vi "ecg_ncs_v2_2Prod_1Cons.vi"() -> ()   [LabVIEW 2016]
uses:
  <instrlib>/niUSRP/niUSRP Timestamp.ctl
  C:/Program Files/National Instruments/LabVIEW 2016/examples/Instrument IO/Serial/support/Serial - Settings.ctl
  <vilib>/Analysis/coordinate.llb/Wrap Angle (array).vi
  <instrlib>/niUSRP/niUSRP Configure Time Start Trigger.vi
  <vilib>/Instr/_visa.llb/VISA Configure Serial Port (Instr).vi
  <vilib>/Analysis/3filter.llb/Butterworth Filter (DBL).vi
  <instrlib>/niUSRP/niUSRP Write Tx Data (2D CDB).vi
  <instrlib>/niUSRP/niUSRP Fetch Rx Data (2D CDB).vi
  <vilib>/measure/NI_MABase.lvlib
  <vilib>/Analysis/NI_AALBase.lvlib
  <vilib>/Analysis/NI_AALPro.lvlib
  <vilib>/Analysis/NI_AAL_Angle.lvlib
panel:
  in  "timeout in ms (-1)":i32=1
  out "size(s) 3":i32
  out "size(s) 2":i32
  out "Serial Settings:Number of Bytes at Serial Port":u32
  in  "Stop":bool
  out "Poor Sensor Quality: \nSensor off":bool
  out "Poor Sensor Quality: \nSensor on":bool
  out "Heart Rate 2":u16[](array[numeric])
  out "Stop Loop":bool=TRUE
  out "Loop index":i32
  out "size(s)":i32
  in  "Read Count":u32=80
  out "return count":u32=24
  in  "Serial Settings":T1={"baud rate"=57600, "data bits"=8, "parity"=enum."None", "stop bits"=10, "flow control"=0} {"flow control" items=["None"=0, "XON/XOFF"=1, "RTS/CTS"=2, "DTR/DSR"=4]; "stop bits" items=["1.0"=10, "1.5"=15, "2.0"=20]; "data bits" min=5 max=8 step=1; "baud rate" items=["75"=75, "110"=110, "134"=134, "150"=150, "300"=300, "600"=600, "1200"=1200, "1800"=1800, "2400"=2400, "4800"=4800, "7200"=7200, "9600"=9600, "14400"=14400, "19200"=19200, "28800"=28800, "38400"=38400, "56000"=56000, "57600"=57600, "115200"=115200, "128000"=128000, "230400"=230400]}
  in  "VISA resource name":refnum<visa-resource-name>="bmd101"
  in  "?":enum32{"ECG", "Heart Rate"}(tab)
  out "?":i16(graph)=106
  out "?":u8[](graph)
  in  "File Name":string="Test"
  in  "order1":i32=5
  in  "Path":path=path "D:/Research/SummerFall17Spring18/CnC/NCS/EcgNcsCorrelation"
  in  "Low-Pass Freq":dbl=200.0 format="%#_13g"
  in  "Sampling Rate":i32=512
  out "Gain":dbl=-15.0
  out "Bandwidth":dbl=56000000.0
  out "Coerced Carrier Frequency":dbl=2000000000.0 format="%#.17g"
  out "Coerced Tx IQ rate":dbl=992969.6965345087
  out "Coerced Rx IQ rate":dbl=1023999.9995512121
  out "error IO":errorcluster={"status"=FALSE, "code"=-1074118647, "source"=""}
  in  "Rx Number of Samples":i32=2000
  in  "Tab Control 2":enum32{"NI-294x/295x", "NI-2900/2901"}(tab)=enum."NI-2900/2901"
  in  "channel 0 carrier\n frequency [Hz]":dbl=2000000000.0 format="%#_6p"
  in  "Rx carrier frequency [Hz]":dbl=2000000000.0 format="%#_6p"
  in  "Tx carrier frequency [Hz]":dbl=1000000000.0 format="%#_6p"
  in  "Start Trigger Time":T2={"whole seconds"=1, "fractional seconds"=0.0}
  out "Tx Active Antenna":string="TX1"
  in  "Tab Control":T3(tab)=enum."Tx"
  out "NCS tag Amp":dbl[](graph)=[6.575627577749796e-12]
  out "NCS tag Phase":dbl[](graph)=[1.1196377624414358e-07]
  out "IQ":dbl[][](graph)=[[-0.008331551052877154], [0.0]]
  out "Tag Amp":dbl[](graph)=[0.008331551052877154]
  out "Tag Phase":dbl[](graph)=[337.4998459209021]
  out "Tx Waveform Graph":waveform(dbl)[](graph)
  in  "Channel 0\nTone Amplitude":dbl=0.707 step=0.05 format="%#.6g"
  in  "Channel 0 \nTone Frequency":dbl=5000.0 format="%#_6p"
  in  "Waveform Size":dbl=2000.0
  in  "Rx Active Antenna":string="RX2"
  in  "Device Name":refnum<k15>="MyB200"
  in  "Tx Gain":dbl=28.0 format="%#_6f"
  in  "Tx IQ Rate":dbl=1000000.0 format="%#_6p"
  in  "Rx Gain":dbl=32.0 format="%#_6f"
  in  "Rx IQ Rate":dbl=1000000.0 format="%#_6p"
  # "Rx Settings"
  # "Tx Settings"
  # "Note that on the NI-2900 and NI-2901, both Rx channels share an LO and both Tx channels share an LO. However, on the NI-294x/295x devices, Rx and Tx of channel 0 share an LO and Rx and Tx of channel 1 share an LO."
  # "This Tx graph should always have end and start tied up since this is being sent in a loop continuously. Otherwise phase jumps will be noticed."
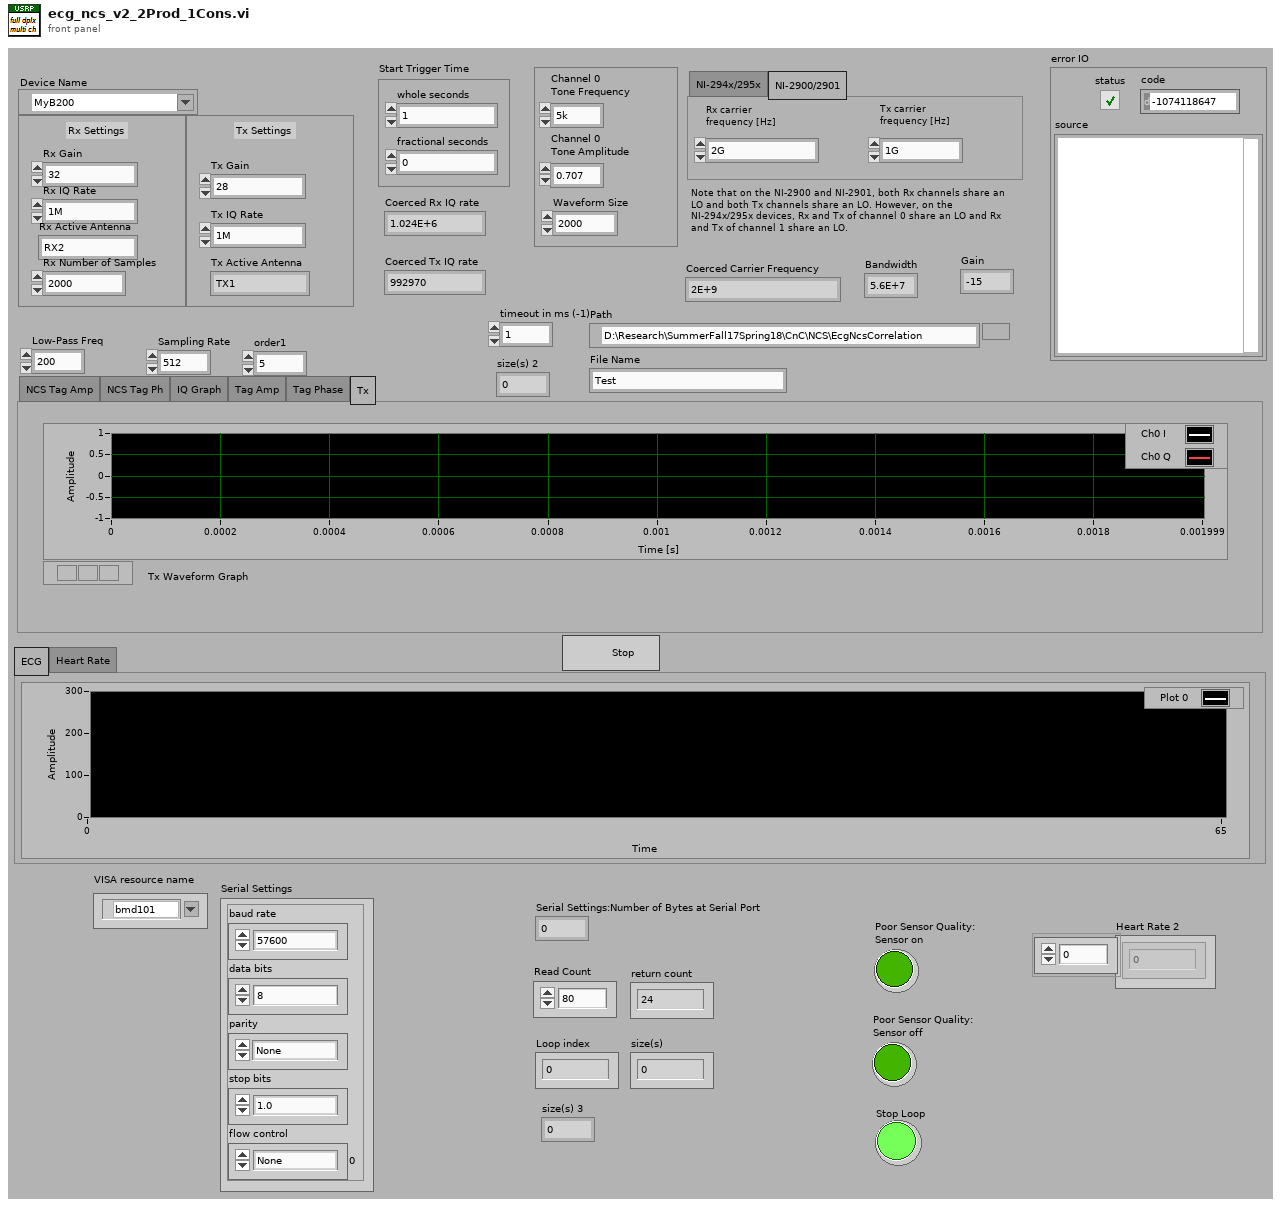
[diagram p1: front panel]
types:
  T1 = typedef "Serial - Settings.ctl" = cluster{"baud rate":u32, "data bits":u16, "parity":enum16{"None", "Odd", "Even", "Mark", "Space"}, "stop bits":u16, "flow control":u16}
  T2 = typedef "niUSRP Timestamp.ctl" = cluster{"whole seconds":u64, "fractional seconds":dbl}
  T3 = enum32{"NCS Tag Amp", "NCS Tag Ph", "IQ Graph", "Tag Amp", "Tag Phase", "Tx"}
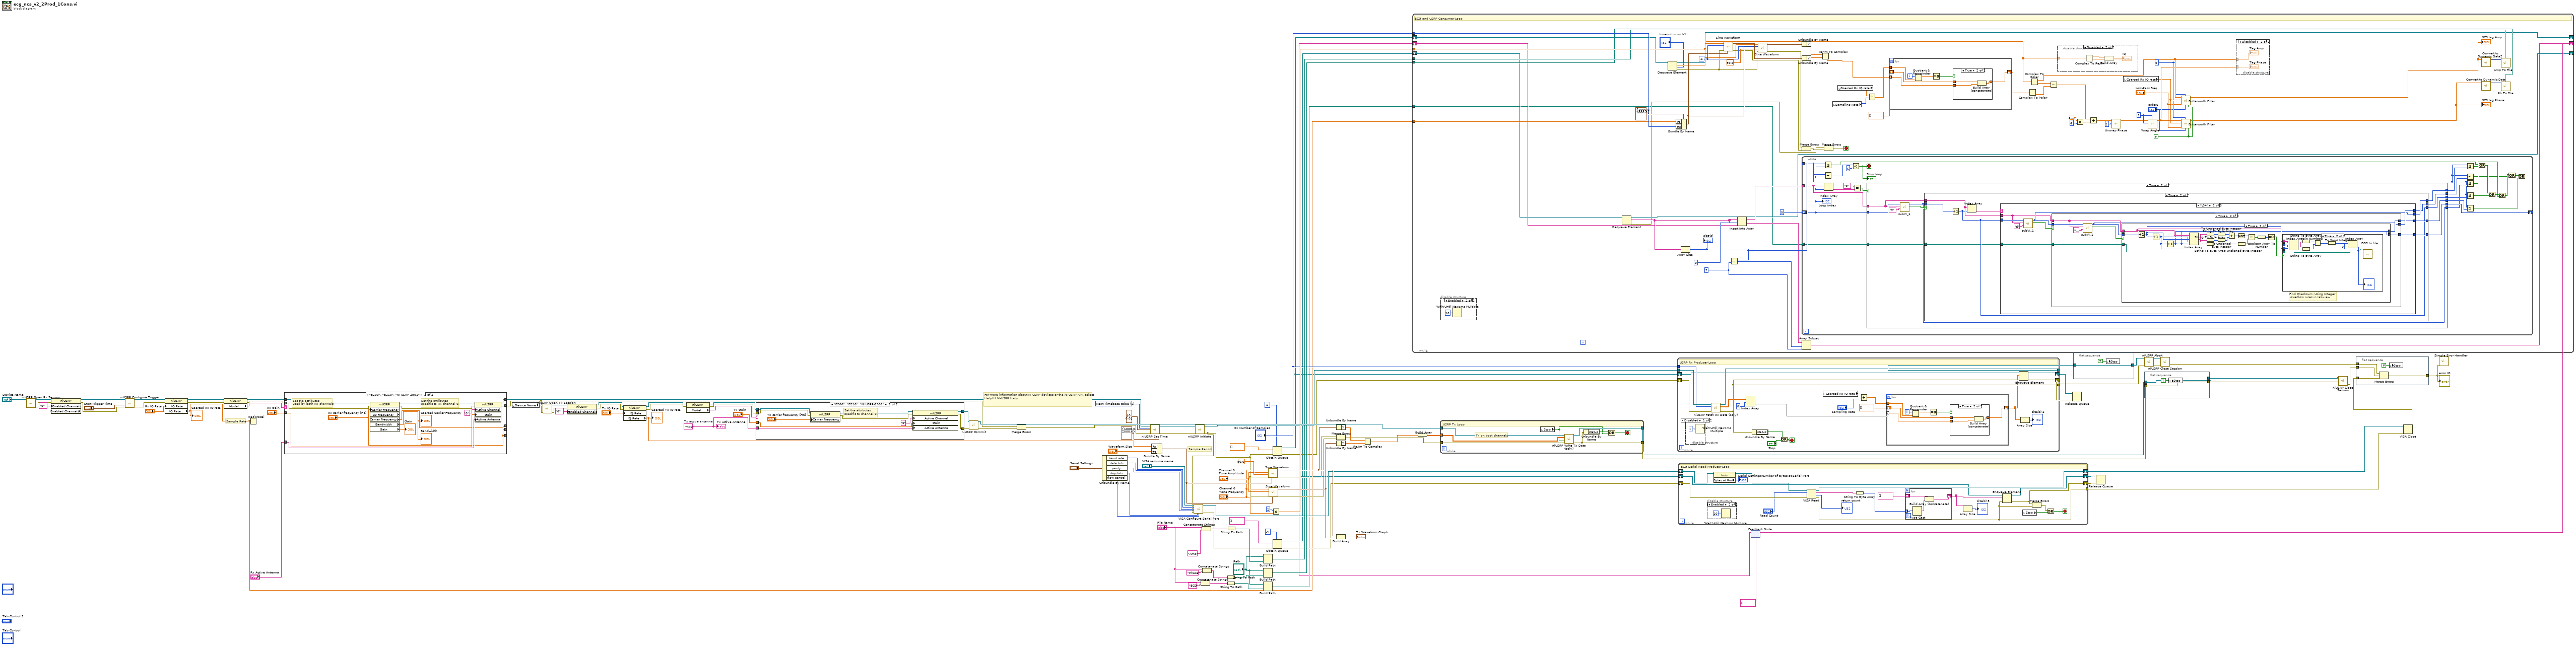
[diagram p0: block diagram]
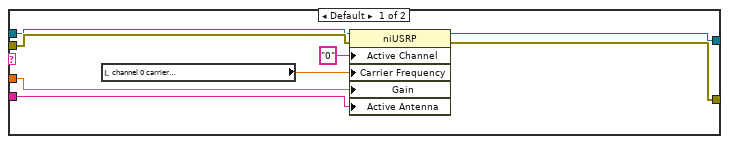
[diagram p5: hidden frame]
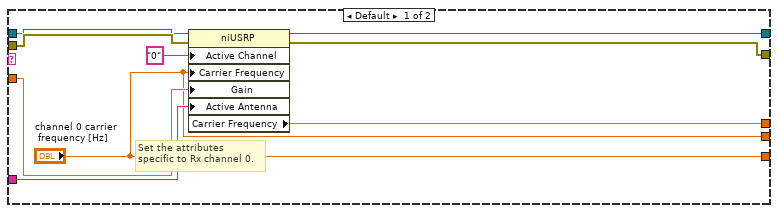
[diagram p6: hidden frame]
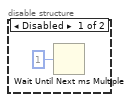
[diagram p7: hidden frame]
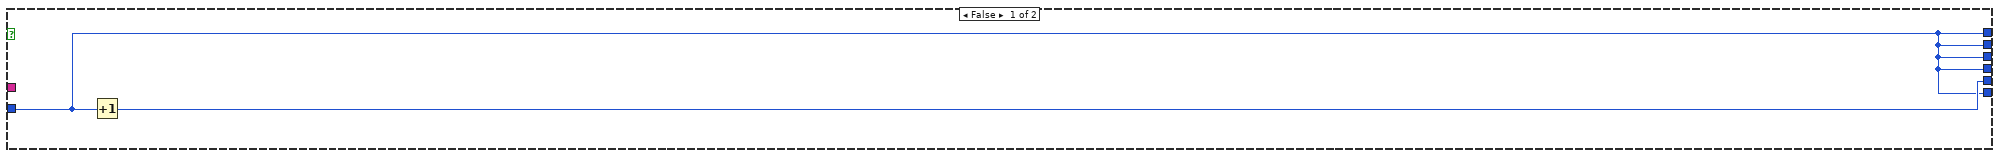
[diagram p9: hidden frame]
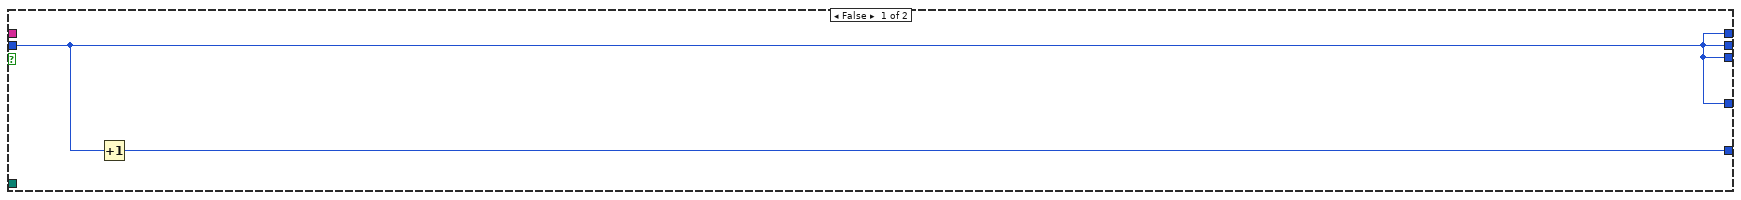
[diagram p10: hidden frame]
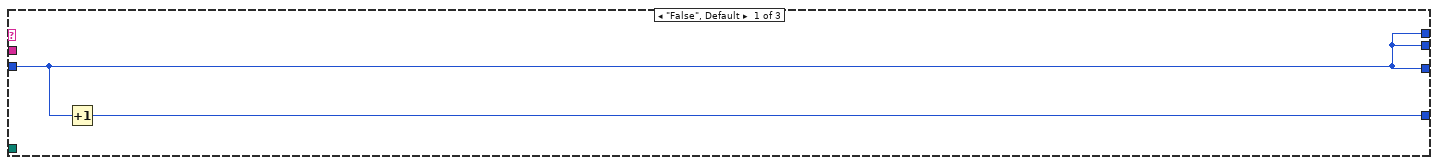
[diagram p11: hidden frame]
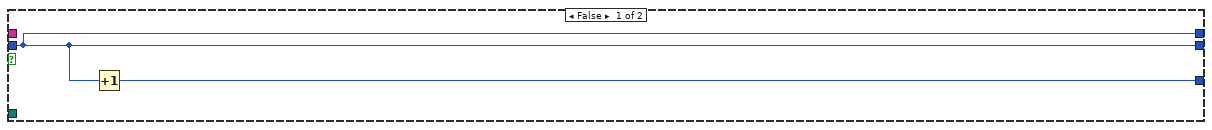
[diagram p12: hidden frame]
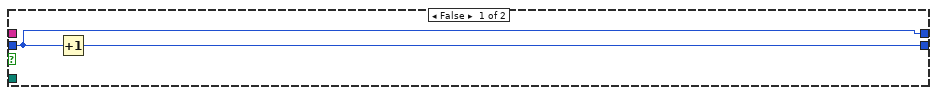
[diagram p13: hidden frame]
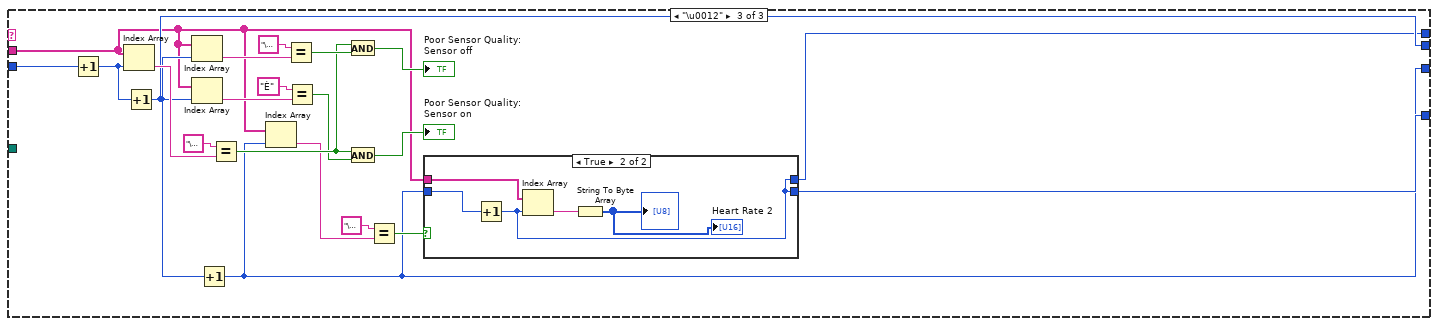
[diagram p15: hidden frame]
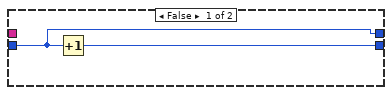
[diagram p16: hidden frame]
diagram:
  w93 = 1 items=["Now", "Next Timebase Edge"] ("apply timestamp")
  w62 = "TX1"  # Tx active antenna
  # "Sample Rate"
  # "Sample Period"
  # "For more information about NI USRP devices or the NI-USRP API, select Help>>NI-USRP Help."
  n1 = call <instrlib>:"niUSRP Open Rx Session.vi"("device names"="Device Name") -> ("session handle out"=w92:refnum<k15>, "error out"=w91:errorcluster)  [unwired: 13 in]
  n2 = property class="niUSRP" props=["Enabled Channels", "Enabled Channels"](reference=w92, error in=w91, "Enabled Channels"="0" ("Configuration:Enabled Channels")) -> (reference out=w90:refnum<k15>, error out=w89:errorcluster)  [unwired: 1 out]
  n3 = call-poly <instrlib>:"niUSRP Configure Trigger.vi"("session handle"=w90, "start trigger time"="Start Trigger Time", "error in (no error)"=w89) -> ("session handle out"=w86:refnum<k15>, "error out"=w85:errorcluster)  [unwired: 11 in]
  n4 = property class="niUSRP"(reference=w86, error in=w85, "IQ Rate"="Rx IQ Rate") -> (reference out=w82:refnum<k15>, error out=w83:errorcluster, "IQ Rate"=w16:dbl)
  "Coerced Rx IQ rate" <- w16
  n5 = property class="niUSRP"(reference=w82, error in=w83) -> (reference out=w77:refnum<k15>, error out=w78:errorcluster, "Model"=w79:string)
  n6 = Reciprocal(x=w16) -> ()  [unwired: 1 out]
  n7 = case shown="\"B200\", \"B210\", \"NI USRP-2901\"" w79 {
    tunnel: w78 -> [w126 w136]
    tunnel: w77 -> [w125 w137]
    tunnel: [w122 w133] -> w81
    tunnel: [w121 w132] -> w80
    tunnel: "Rx Gain" -> [w124 w139]
    tunnel: "Rx Active Antenna" -> [w123 w138]
    tunnel: [w119 w128] -> _
    tunnel: ["channel 0 carrier\n frequency [Hz]" "Rx carrier frequency [Hz]"] -> _
    tunnel: ["channel 0 carrier\n frequency [Hz]" "Rx carrier frequency [Hz]"] -> _
    frame Default {
      # "Set the attributes \nspecific to Rx channel 0."
      n8 = property class="niUSRP"(reference=w125, error in=w126, "Active Channel"="0", "Carrier Frequency"="channel 0 carrier\n frequency [Hz]", "Gain"=w124, "Active Antenna"=w123) -> (reference out=w122:refnum<k15>, error out=w121:errorcluster, "Carrier Frequency"=w119:dbl)
    }
    frame "B200", "B210", "NI USRP-2901" {
      # "Set the attributes \nused by both Rx channels"
      # "Set the attributes \nspecific to Rx channel 0."
      n9 = property class="niUSRP" props=["Carrier Frequency", "LO Frequency", "Carrier Frequency", "Bandwidth", "Gain"](reference=w137, error in=w136, "Carrier Frequency"="Rx carrier frequency [Hz]") -> (reference out=w135:refnum<k15>, error out=w134:errorcluster, "Carrier Frequency"=w128:dbl, "Bandwidth"=→"Bandwidth":dbl, "Gain"=→"Gain":dbl)  [unwired: 1 out]
      "Coerced Carrier Frequency" <- w128
      n10 = property class="niUSRP"(reference=w135, error in=w134, "Active Channel"="0", "Gain"=w139, "Active Antenna"=w138) -> (reference out=w133:refnum<k15>, error out=w132:errorcluster)
    }
  }
  n11 = local read "Device Name"() -> (w113:refnum<k15>)
  n12 = call <instrlib>:"niUSRP Open Tx Session.vi"("device names"=w113, "error in (no error)"=w80) -> ("session handle out"=w88:refnum<k15>, "error out"=w87:errorcluster)  [unwired: 12 in]
  n13 = property class="niUSRP"(reference=w88, error in=w87, "Enabled Channels"="0" ("Configuration:Enabled Channels")) -> (reference out=w74:refnum<k15>, error out=w73:errorcluster)
  n14 = property class="niUSRP"(reference=w74, error in=w73, "IQ Rate"="Tx IQ Rate") -> (reference out=w68:refnum<k15>, error out=w69:errorcluster, "IQ Rate"=w66:dbl)
  "Coerced Tx IQ rate" <- w66
  n15 = property class="niUSRP"(reference=w68, error in=w69) -> (reference out=w70:refnum<k15>, error out=w71:errorcluster, "Model"=w67:string)
  n16 = case shown="\"B200\", \"B210\", \"NI USRP-2901\"" w67 {
    tunnel: "Tx Gain" -> [w148 w158]
    tunnel: w62 -> [w146 w156]
    tunnel: [w142 w150] -> w64
    tunnel: [w141 w149] -> w65
    tunnel: w71 -> [w145 w152]
    tunnel: w70 -> [w144 w155]
    frame Default {
      n17 = local read "channel 0 carrier\n frequency [Hz]"() -> (w143:dbl)
      n18 = property class="niUSRP"(reference=w144, error in=w145, "Active Channel"="0", "Carrier Frequency"=w143, "Gain"=w148, "Active Antenna"=w146) -> (reference out=w142:refnum<k15>, error out=w141:errorcluster)
    }
    frame "B200", "B210", "NI USRP-2901" {
      # "Set the attributes \nspecific to channel 0."
      n19 = property class="niUSRP"(reference=w155, error in=w152, "Carrier Frequency"="Tx carrier frequency [Hz]") -> (reference out=w154:refnum<k15>, error out=w153:errorcluster)
      n20 = property class="niUSRP"(reference=w154, error in=w153, "Active Channel"="0", "Gain"=w158, "Active Antenna"=w156) -> (reference out=w150:refnum<k15>, error out=w149:errorcluster)
    }
  }
  n21 = call <instrlib>:"niUSRP Commit.vi"("session handle"=w64, "error in (no error)"=w65) -> ("session handle out"=w115:refnum<k15>, "error out"=w116:errorcluster)  [unwired: 12 in]
  n22 = Merge Errors(w80, w116) -> (w95:errorcluster)
  n23 = Unbundle By Name("Serial Settings") -> ("baud rate"=w23:u32, "data bits"=w24:u16, "parity"=w25:enum16{"None", "Odd", "Even", "Mark", "Space"}, "stop bits"=w26:u16, "flow control"=w27:u16)
  n24 = call <instrlib>:"niUSRP Set Time.vi"("session handle"=w81, "apply timestamp"=w93, "timestamp"=T2 {"whole seconds"=0, "fractional seconds"=0.0}, "error in (no error)"=w95) -> ("session handle out"=w97:refnum<k15>, "error out"=w96:errorcluster)  [unwired: 10 in]
  n25 = Bundle By Name(cluster=cluster{"Fs":dbl, "#s":dbl} {"Fs"=1000.0, "#s"=1000.0} ("sampling info"), "Fs"=w66, "#s"="Waveform Size") -> (w99:cluster{"Fs":dbl, "#s":dbl})
  n26 = call <instrlib>:"niUSRP Initiate.vi"("session handle"=w97, "error in (no error)"=w96) -> ("session handle out"=w19:refnum<k15>, "error out"=w5:errorcluster)  [unwired: 12 in]
  n27 = call-poly "VISA Configure Serial Port"("VISA resource name"="VISA resource name", "baud rate (9600)"=w23, "data bits (8)"=w24, "parity (0:none)"=w25, "error in (no error)"=w5, "stop bits (10: 1 bit)"=w26, "flow control (0:none)"=w27) -> ("VISA resource name out"=w28:refnum<visa-resource-name>, "error out"=w6:errorcluster)  [unwired: 3 in, 4 out]
  n28 = Concatenate Strings("File Name", "ECG") -> (w36:string)
  n29 = Concatenate Strings("File Name", "Amp") -> (w46:string)
  n30 = Concatenate Strings("File Name", "Phase") -> (w43:string)
  n31 = String To Path(string=w43) -> (path=w42:path)
  n32 = String To Path(string=w36) -> (path=w35:path)
  n33 = String To Path(string=w46) -> (path=w45:path)
  n34 = Build Path(base path="Path", name or relative path=w45) -> (appended path=w48:path)
  n35 = Build Path(base path="Path", name or relative path=w42) -> (appended path=w41:path)
  n36 = Build Path(base path="Path", name or relative path=w35) -> (appended path=w9:path)
  n37 = call <vilib>:"Sine Waveform.vi"("sampling info"=w99, "error in (no error)"=w5, "phase"=90.0, "amplitude"="Channel 0\nTone Amplitude", "frequency"="Channel 0 \nTone Frequency") -> ("error out"=w60:errorcluster, "signal out"=w107:waveform(dbl))  [unwired: 5 in]
  n38 = call <vilib>:"Sine Waveform.vi"("sampling info"=w99, "error in (no error)"=w5, "amplitude"="Channel 0\nTone Amplitude", "frequency"="Channel 0 \nTone Frequency") -> ("error out"=w61:errorcluster, "signal out"=w108:waveform(dbl))  [unwired: 6 in]
  n39 = Multiply(x=2, y="Channel 0 \nTone Frequency") -> (x*y=w49:dbl)
  n40 = Obtain Queue(max queue size (-1, unlimited)=-1, element data type=dbl[] [], error in (no error)=w5) -> (queue out=w11:refnum<queue>, error out=w15:errorcluster)  [unwired: 2 in, 1 out]
  n41 = Obtain Queue(max queue size (-1, unlimited)=-1, element data type=string[] [], error in (no error)=w6) -> (queue out=w8:refnum<queue>, error out=w30:errorcluster)  [unwired: 2 in, 1 out]
  n42 = Unbundle By Name(w107) -> ("Y"=w106:dbl[])
  n43 = Merge Errors(w60, w61) -> (w59:errorcluster)
  n44 = Unbundle By Name(w108) -> ("Y"=w105:dbl[])
  n45 = Build Array(w107, w108) -> (→"Tx Waveform Graph":waveform(dbl)[])
  n46 = Re/Im To Complex(1:w105, 2:w106) -> (0:w101:cdb[])
  n47 = Build Array(w101) -> (w100:cdb[][])
  n48 = while {
    tunnel: w115 -> [w166]
    tunnel: w59 -> [w165]
    tunnel: [w163] -> w58
    tunnel: [w161] -> w54
    tunnel: w100 -> [w160]
    stop <- w162 stop-if-true
    # "Tx on both channels"
    # "USRP Tx Loop"
    n49 = local read "Stop"() -> (w159:bool)
    n50 = call-poly <instrlib>:"niUSRP Write Tx Data (poly).vi"("session handle"=w166, "data"=w160, "end of data?"=w159, "error in (no error)"=w165) -> ("session handle out"=w161:refnum<k15>, "error out"=w163:errorcluster)  [unwired: 10 in]
    n51 = Unbundle By Name(w163) -> ("status"=w164:bool)
    n52 = Compound Arithmetic op=OR(w164, w159) -> (w162:bool)
  }
  n53 = while {
    tunnel: w19 -> [w185]
    tunnel: [w184] -> w18
    tunnel: "Rx Number of Samples" -> [w183]
    tunnel: [w177] -> w10
    shift-right: [w180] -> w13
    shift-left: w11 -> [w181]
    shift-right: [w179] -> w12
    shift-left: w15 -> [w178]
    stop <- w182 stop-if-true
    # "USRP Rx Producer Loop"
    n54 = disable-structure shown="Disabled" {
      frame Disabled {
        n55 = Wait Until Next ms Multiple(millisecond multiple=u32 1 ("milliseconds to wait")) -> ()  [unwired: 1 out]
      }
      frame Enabled {
      }
    }
    n56 = call-poly <instrlib>:"niUSRP Fetch Rx Data (poly).vi"("session handle"=w185, "number of samples"=w183, "error in (no error)"=w178) -> ("session handle out"=w184:refnum<k15>, "data"=w175:cdb[][], "error out"=w177:errorcluster)  [unwired: 9 in, 1 out]
    n57 = Index Array(array=w175, index (row)=0 ("y")) -> (element=w169:cdb[])  [unwired: 1 in]
    n58 = Unbundle By Name(w177) -> ("status"=w186:bool)
    n59 = Or(x=w186, y="Stop") -> (x .or. y?=w182:bool)
    n60 = local read "Coerced Rx IQ rate"() -> (w173:dbl)
    n61 = Divide(x=w173, y="Sampling Rate") -> (x/y=w171:dbl)
    n62 = for {
      tunnel: w169 -> [w193] mode=indexing
      shift-right: [w191] -> w168
      shift-left: dbl[] [] -> [w192]
      tunnel: w171 -> [w187]
      i -> [w190]
      n63 = Quotient & Remainder(x=w190, y=w187) -> (x-y*floor(x/y)=w188:dbl)  [unwired: 1 out]
      n64 = Equal To 0?(x=w188) -> (x = 0?=w189:bool)
      n65 = case shown="True" w189 {
        tunnel: w193 -> [_ w197]
        tunnel: w192 -> [w194 w196]
        tunnel: [w194 w195] -> w191
        frame False {
        }
        frame True {
          n66 = Build Array (concatenate)(w196, w197) -> (w195:cdb[])
        }
      }
    }
    n67 = Enqueue Element(queue=w181, element=w168, error in (no error)=w177) -> (queue out=w180:refnum<queue>, error out=w179:errorcluster)  [unwired: 1 in, 1 out]
    n68 = Array Size(array=w168) -> (size(s)=→"size(s) 2":i32)
  }
  n69 = while {
    shift-right: [w215] -> w33
    shift-left: w28 -> [w206]
    tunnel: [w207] -> w34
    shift-right: [w211] -> w32
    shift-left: w30 -> [w208]
    shift-right: [w212] -> w31
    shift-left: w8 -> [w213]
    stop <- w217 stop-if-true
    # "ECG Serial Read Producer Loop"
    n70 = disable-structure shown="Enabled" {
      frame Disabled {
      }
      frame Enabled {
        n71 = Wait Until Next ms Multiple(millisecond multiple=u32 10) -> ()  [unwired: 1 out]
      }
    }
    n72 = property class="Instr"(reference=w206) -> (reference out=w205:refnum<visa-resource-name>, "Bytes at Port"=→"Serial Settings:Number of Bytes at Serial Port":u32)  [unwired: 1 in, 1 out]
    n73 = VISA Read(VISA resource name=w205, byte count="Read Count", error in (no error)=w208) -> (VISA resource name out=w215:refnum<visa-resource-name>, read buffer=w204:string, return count=→"return count":u32, error out=w207:errorcluster)
    n74 = String To Byte Array(string=w204) -> (unsigned byte array=w214:u8[])
    n75 = for {
      tunnel: w214 -> [w222] mode=indexing
      shift-right: [w219] -> w202
      shift-left: string[] [] -> [w220]
      n76 = Type Cast(x=w222) -> (*(type *) &x=w221:string)  [unwired: 1 in]
      n77 = Build Array (concatenate)(w220, w221) -> (w219:string[])
    }
    n78 = Array Size(array=w202) -> (size(s)=→"size(s) 3":i32)
    n79 = Enqueue Element(queue=w213, element=w202, error in (no error)=w207) -> (queue out=w212:refnum<queue>, error out=w211:errorcluster)  [unwired: 1 in, 1 out]
    n80 = local read "Stop"() -> (w209:bool)
    n81 = Merge Errors(w211, w207) -> (w210:errorcluster)
    n82 = Or(x=w210, y=w209) -> (x .or. y?=w217:bool)
  }
  n83 = feedback #1(string[] []) -> (w2:string[])
  n84 = while {
    tunnel: "Rx Number of Samples" -> [w282]
    tunnel: w16 -> [w274]
    tunnel: w49 -> [w275]
    tunnel: w48 -> [w273]
    tunnel: w41 -> [w253]
    shift-right: [w249] -> _
    shift-left: w11 -> [w250]
    tunnel: w9 -> [w223]
    shift-right: [w241] -> _
    shift-left: w8 -> [w242]
    shift-right: [w238] -> w7
    shift-left: w2 -> [w237]
    stop <- w240 stop-if-true
    w246 = 7
    w262 = 2 ("y")
    w255 = TRUE
    w257 = 0
    w280 = -1
    # "ECG and USRP Consumer Loop"
    n85 = disable-structure shown="Enabled" {
      frame Disabled {
        n86 = Wait Until Next ms Multiple(millisecond multiple=u32 1) -> ()  [unwired: 1 out]
      }
      frame Enabled {
        n87 = Wait Until Next ms Multiple(millisecond multiple=u32 10) -> ()  [unwired: 1 out]
      }
    }
    n88 = Dequeue Element(queue=w242) -> (queue out=w241:refnum<queue>, element=w239:string[], error out=w234:errorcluster)  [unwired: 2 in, 1 out]
    n89 = Dequeue Element(queue=w250, timeout in ms (-1)="timeout in ms (-1)") -> (queue out=w249:refnum<queue>, element=w233:dbl[], error out=w236:errorcluster)  [unwired: 1 in, 1 out]
    n90 = Bundle By Name(cluster=cluster{"Fs":dbl, "#s":dbl} {"Fs"=1000.0, "#s"=1000.0} ("sampling info"), "Fs"=w274, "#s"=w282) -> (w279:cluster{"Fs":dbl, "#s":dbl})
    n91 = Array Size(array=w239) -> (size(s)=w244:i32)
    "size(s)" <- w244
    n92 = call <vilib>:"Sine Waveform.vi"("sampling info"=w279, "error in (no error)"=w236, "amplitude"=w280, "frequency"=w275) -> ("error out"=w278:errorcluster, "signal out"=w283:waveform(dbl))  [unwired: 6 in]
    n93 = Subtract(x=w244, y=w246) -> (x-y=w245:i32)
    n94 = Insert Into Array(array=w239, index=0, new element=w237) -> (w247:string[])
    n95 = call <vilib>:"Sine Waveform.vi"("sampling info"=w279, "error in (no error)"=w236, "phase"=90.0, "amplitude"=w280, "frequency"=w275) -> ("error out"=w277:errorcluster, "signal out"=w276:waveform(dbl))  [unwired: 5 in]
    n96 = Unbundle By Name(w276) -> ("Y"=w271:dbl[])
    n97 = Unbundle By Name(w283) -> ("Y"=w270:dbl[])
    n98 = Merge Errors(w277, w278) -> (w235:errorcluster)
    n99 = while {
      tunnel: w247 -> [w319]
      shift-right: [w323] -> _
      shift-left: 0 -> [w302]
      tunnel: w244 -> [w303]
      tunnel: w223 -> [w298]
      stop <- w299 stop-if-true
      n100 = Less Or Equal?(x=w303, y=w302) -> (x <= y?=w304:bool)
      n101 = Subtract(x=w303, y=w302) -> (x-y=w301:i32)
      n102 = Index Array(array=w319, index=w302) -> (element=w322:string)
      n103 = Less?(x=w301, y=6) -> (x < y?=w299:bool)
      "Stop Loop" <- w299
      n104 = Equal?(x="ª", y=w322) -> (x = y?=w320:bool)
      n105 = case shown="True" w320 {
        tunnel: w302 -> [w324 w335]
        tunnel: [w325 w333] -> w323
        tunnel: w319 -> [_ w327]
        tunnel: [w324 w332] -> w318
        tunnel: [w324 w331] -> w316
        tunnel: [w324 w330] -> w313
        tunnel: [w324 w329] -> w310
        tunnel: [w324 w328] -> w307
        tunnel: w298 -> [_ w326]
        frame False {
          n106 = Increment(x=w324) -> (x+1=w325:i32)
        }
        frame True {
          n107 = call "subVI_1.vi"("String"="ª", "Array"=w327, "Numeric in"=w335) -> ("Boolean"=w334:bool, "Numeric out"=w332:i32)  [unwired: 7 in]
          n108 = case shown="True" w334 {
            tunnel: w332 -> [w337 w341]
            tunnel: [w338 w347] -> w333
            tunnel: w327 -> [_ w346]
            tunnel: [w337 w342] -> w331
            tunnel: [w337 w345] -> w330
            tunnel: [w337 w344] -> w329
            tunnel: [w337 w343] -> w328
            tunnel: w326 -> [_ w339]
            frame False {
              n109 = Increment(x=w337) -> (x+1=w338:i32)
            }
            frame True {
              n110 = Increment(x=w341) -> (x+1=w342:i32)
              n111 = Index Array(array=w346, index=w342) -> (element=w340:string)
              n112 = case shown="\"\\04\"" w340 {
                tunnel: w342 -> [w348 w355 w422]
                tunnel: [w349 w358 w404] -> w347
                tunnel: w346 -> [_ w351 w406]
                tunnel: [w348 w353 w408] -> w345
                tunnel: [w348 w357 w405] -> w344
                tunnel: [w348 w356 w403] -> w343
                tunnel: w339 -> [_ w350 _]
                frame "False", Default {
                  n113 = Increment(x=w348) -> (x+1=w349:i32)
                }
                frame "\u0004" {
                  n114 = call "subVI_1.vi"("String"="€", "Array"=w351, "Numeric in"=w355) -> ("Boolean"=w352:bool, "Numeric out"=w353:i32)  [unwired: 7 in]
                  n115 = case shown="True" w352 {
                    tunnel: w353 -> [w359 w366]
                    tunnel: [w360 w368] -> w358
                    tunnel: w351 -> [_ w365]
                    tunnel: [w359 w363] -> w357
                    tunnel: [w359 w367] -> w356
                    tunnel: w350 -> [_ w361]
                    frame False {
                      n116 = Increment(x=w359) -> (x+1=w360:i32)
                    }
                    frame True {
                      n117 = call "subVI_1.vi"("String"="\u0002", "Array"=w365, "Numeric in"=w366) -> ("Boolean"=w362:bool, "Numeric out"=w363:i32)  [unwired: 7 in]
                      n118 = case shown="True" w362 {
                        tunnel: w363 -> [w369 w375]
                        tunnel: [w370 w372] -> w368
                        tunnel: w365 -> [_ w376]
                        tunnel: [w369 w372] -> w367
                        tunnel: w361 -> [_ w371]
                        frame False {
                          n119 = Increment(x=w369) -> (x+1=w370:i32)
                        }
                        frame True {
                          # "Find Checksum: Using Integer\n overflow rules in labview"
                          n120 = Increment(x=w375) -> (x+1=w374:i32)
                          n121 = Increment(x=w374) -> (x+1=w373:i32)
                          n122 = Increment(x=w373) -> (x+1=w372:i32)
                          n123 = Index Array(array=w376, index #1=w374, index #2=w373, index #3=w372) -> (element #1=w390:string, element #2=w389:string, element #3=w383:string)
                          n124 = String To Byte Array(string=w390) -> (unsigned byte array=w388:u8[])
                          n125 = String To Byte Array(string=w389) -> (unsigned byte array=w387:u8[])
                          n126 = String To Byte Array(string=w383) -> (unsigned byte array=w382:u8[])
                          n127 = To Unsigned Byte Integer(number=w388) -> (unsigned 8bit integer=w386:u8[])
                          n128 = To Unsigned Byte Integer(number=w387) -> (unsigned 8bit integer=w385:u8[])
                          n129 = Add(x=w386, y=w385) -> (x+y=w384:u8[])
                          n130 = Not(x=w384) -> (.not. x?=w381:u8[])
                          n131 = To Unsigned Byte Integer(number=w382) -> (unsigned 8bit integer=w380:u8[])
                          n132 = Equal?(x=w381, y=w380) -> (x = y?=w379:bool[])
                          n133 = Boolean Array To Number(Boolean array=w379) -> (number=w378:u32)
                          n134 = Equal To 0?(x=w378) -> (x = 0?=w377:bool)
                          n135 = case shown="True" w377 {
                            tunnel: w376 -> [_ w402]
                            tunnel: w374 -> [_ w396]
                            tunnel: w373 -> [_ w395]
                            tunnel: w371 -> [_ w392]
                            frame False {
                            }
                            frame True {
                              n136 = Index Array(array=w402, index #1=w396, index #2=w395) -> (element #1=w401:string, element #2=w400:string)
                              n137 = String To Byte Array(string=w401) -> (unsigned byte array=w399:u8[])
                              n138 = String To Byte Array(string=w400) -> (unsigned byte array=w398:u8[])
                              n139 = Join Numbers(hi=w399, lo=w398) -> ((hi.lo)=w397:u16[])
                              n140 = To Word Integer(number=w397) -> (16bit integer=w394:i16[])
                              n141 = Index Array(array=w394, index=0) -> (element=w391:i16)
                              "?" <- w391
                              n142 = call "ECG to file"("Signals"=w391, "Filename"=w392) -> ()  [unwired: 15 in, 3 out]
                            }
                          }
                        }
                      }
                    }
                  }
                }
                frame "\u0012" {
                  n143 = Increment(x=w422) -> (x+1=w418:i32)
                  n144 = Index Array(array=w406, index=w418) -> (element=w421:string)
                  n145 = Increment(x=w418) -> (x+1=w408:i32)
                  n146 = Index Array(array=w406, index=w408) -> (element=w419:string)
                  n147 = Index Array(array=w406, index=w408) -> (element=w416:string)
                  n148 = Increment(x=w408) -> (x+1=w403:i32)
                  n149 = Equal?(x="\u0002", y=w421) -> (x = y?=w413:bool)
                  n150 = Index Array(array=w406, index=w403) -> (element=w409:string)
                  n151 = Equal?(x="\u0000", y=w419) -> (x = y?=w415:bool)
                  n152 = Equal?(x="È", y=w416) -> (x = y?=w412:bool)
                  n153 = And(x=w413, y=w415) -> (x .and. y?=→"Poor Sensor Quality: \nSensor off":bool)
                  n154 = And(x=w413, y=w412) -> (x .and. y?=→"Poor Sensor Quality: \nSensor on":bool)
                  n155 = Equal?(x="\u0003", y=w409) -> (x = y?=w407:bool)
                  n156 = case shown="True" w407 {
                    tunnel: w403 -> [w424 w430]
                    tunnel: w406 -> [_ w429]
                    tunnel: [w424 w428] -> w405
                    tunnel: [w425 w428] -> w404
                    frame False {
                      n157 = Increment(x=w424) -> (x+1=w425:i32)
                    }
                    frame True {
                      n158 = Increment(x=w430) -> (x+1=w428:i32)
                      n159 = Index Array(array=w429, index=w428) -> (element=w427:string)
                      n160 = String To Byte Array(string=w427) -> (unsigned byte array=→"Heart Rate 2" →"?":u8[])
                    }
                  }
                }
              }
            }
          }
        }
      }
      n161 = Less Or Equal?(x=w303, y=w313) -> (x <= y?=w311:bool)
      n162 = Less Or Equal?(x=w303, y=w310) -> (x <= y?=w308:bool)
      n163 = Less Or Equal?(x=w303, y=w318) -> (x <= y?=w317:bool)
      n164 = Less Or Equal?(x=w303, y=w316) -> (x <= y?=w314:bool)
      n165 = Less Or Equal?(x=w303, y=w307) -> (x <= y?=w305:bool)
      n166 = Or(x=w304, y=w317) -> (x .or. y?=w315:bool)
      n167 = Or(x=w315, y=w314) -> (x .or. y?=w312:bool)
      n168 = Or(x=w312, y=w311) -> (x .or. y?=w309:bool)
      n169 = Or(x=w309, y=w308) -> (x .or. y?=w306:bool)
      n170 = Or(x=w306, y=w305) -> ()  [unwired: 1 out]
      "Loop index" <- w302
    }
    n171 = Array Subset(array=w239, index=w245, length=w246) -> (w238:string[])
    n172 = Re/Im To Complex(1:w270, 2:w271) -> (0:w229:cdb[])
    n173 = Merge Errors(w234, w235) -> (w240:errorcluster)
    n174 = local read "Sampling Rate"() -> (w227:i32)
    n175 = local read "Coerced Rx IQ rate"() -> (w231:dbl)
    n176 = Divide(x=w231, y=w227) -> (x/y=w230:dbl)
    n177 = for {
      tunnel: w229 -> [w293] mode=indexing
      shift-right: [w291] -> w228
      shift-left: dbl[] [] -> [w292]
      tunnel: w230 -> [w287]
      i -> [w290]
      n178 = Quotient & Remainder(x=w290, y=w287) -> (x-y*floor(x/y)=w288:dbl)  [unwired: 1 out]
      n179 = Equal To 0?(x=w288) -> (x = 0?=w289:bool)
      n180 = case shown="True" w289 {
        tunnel: w293 -> [_ w297]
        tunnel: w292 -> [w294 w296]
        tunnel: [w294 w295] -> w291
        frame False {
        }
        frame True {
          n181 = Build Array (concatenate)(w296, w297) -> (w295:cdb[])
        }
      }
    }
    n182 = Complex To Polar(r * e^(i*theta)=w228) -> (theta=w265:dbl[])  [unwired: 1 out]
    n183 = Complex To Polar(r * e^(i*theta)=w233) -> (r=w272:dbl[], theta=w260:dbl[])
    n184 = Subtract(x=w260, y=w265) -> (x-y=w264:dbl[])
    n185 = disable-structure shown="Disabled" {
      disable-tunnel: w233 -> [_ w433]
      frame Enabled {
      }
      frame Disabled {
        n186 = Complex To Re/Im(x + iy=w433) -> (x=w436:dbl[], y=w435:dbl[])
        n187 = Build Array(w436, w435) -> (→"IQ":dbl[][])
      }
    }
    n188 = Multiply(x=3.141592653589793, y=6) -> (x*y=w266:dbl)
    n189 = Add(x=w264, y=w266) -> (x+y=w263:dbl[])
    n190 = call <vilib>:"Unwrap Phase.vi"("phase unit"=1 ("y"), "Phase"=w263) -> ("Unwrapped Phase"=w261:dbl[])  [unwired: 8 in, 1 out]
    n191 = local read "Coerced Rx IQ rate"() -> (w258:dbl)
    n192 = call-poly <vilib>:"Wrap Angle.vi"("angle units"=w262, "angle range"=w262, "Angle In"=w261) -> ("Angle Out"=w259:dbl[])  [unwired: 7 in, 1 out]
    n193 = call-poly <vilib>:"Butterworth Filter.vi"("init/cont (init:F)"=w255, "order"="order1", "filter type"=w257, "low cutoff freq: fl"="Low-Pass Freq", "sampling freq: fs"=w258, "X"=w272) -> ("Filtered X"=w226:dbl[])  [unwired: 2 in, 1 out]
    "NCS tag Amp" <- w226
    n194 = call-poly <vilib>:"Butterworth Filter.vi"("init/cont (init:F)"=w255, "order"="order1", "filter type"=w257, "low cutoff freq: fl"="Low-Pass Freq", "sampling freq: fs"=w258, "X"=w259) -> ("Filtered X"=w225:dbl[])  [unwired: 2 in, 1 out]
    "NCS tag Phase" <- w225
    n195 = disable-structure shown="Disabled" {
      disable-tunnel: w272 -> [_ w432]
      disable-tunnel: w259 -> [_ w431]
      frame Enabled {
      }
      frame Disabled {
        "Tag Amp" <- w432
        "Tag Phase" <- w431
      }
    }
    n196 = call "Convert to Dynamic Data2"("Array"=w226) -> ("Dynamic Data Type"=w251:dynamicdata)  [unwired: 3 in]
    n197 = call "Convert to Dynamic Data"("Array"=w225) -> ("Dynamic Data Type"=w254:dynamicdata)  [unwired: 3 in]
    n198 = call "Amp To File"("Signals"=w251, "Filename"=w273) -> ()  [unwired: 15 in, 3 out]
    n199 = call "Ph To File"("Signals"=w254, "Filename"=w253) -> ()  [unwired: 15 in, 3 out]
  }
  n200 = feedback-in #1(w7) -> ()
  n201 = Release Queue(queue=w13, error in (no error)=w12) -> ()  [unwired: 1 in, 3 out]
  n202 = flat-sequence {
    tunnel: [w437] -> w56
    tunnel: w18 -> [w437]
    frame #0 {
      n203 = local write "Stop"(TRUE ("STOP")) -> ()
    }
  }
  n204 = Release Queue(queue=w31, error in (no error)=w32) -> ()  [unwired: 1 in, 3 out]
  n205 = call <instrlib>:"niUSRP Abort.vi"("session handle"=w56, "error in (no error)"=w10) -> ("session handle out"=w112:refnum<k15>, "error out"=w111:errorcluster)  [unwired: 12 in]
  n206 = flat-sequence {
    tunnel: [w440] -> w57
    tunnel: w58 -> [w440]
    tunnel: [w439] -> w55
    tunnel: w54 -> [w439]
    frame #0 {
      n207 = local write "Stop"(TRUE ("STOP")) -> ()
    }
  }
  n208 = call <instrlib>:"niUSRP Close Session.vi"("session handle"=w112, "error in (no error)"=w111) -> ("error out"=w52:errorcluster)  [unwired: 13 in]
  n209 = call <instrlib>:"niUSRP Close Session.vi"("session handle"=w55, "error in (no error)"=w57) -> ("error out"=w53:errorcluster)  [unwired: 13 in]
  n210 = flat-sequence {
    tunnel: w53 -> [w445]
    tunnel: [w444] -> w40
    tunnel: w52 -> [w443]
    tunnel: w20 -> [w442]
    frame #0 {
      n211 = Merge Errors(w443, w445, w442) -> (w444:errorcluster)
      n212 = local write "Stop"(FALSE ("STOP")) -> ()
    }
  }
  n213 = VISA Close(VISA resource name=w33, error in (no error)=w34) -> (error out=w20:errorcluster)
  n214 = call <vilib>:"Simple Error Handler.vi"("error in (no error)"=w40) -> ()  [unwired: 1 in, 8 out]
  "Tx Active Antenna" <- w62
  "error IO" <- w40
